vi "fgv_sound_info.vi"(7 "cmd":T2, 8 "error in (no error)":errorcluster caption="error in", 11 "info":T1) -> (0 "error out":errorcluster, 3 "info out":T1)   [LabVIEW 2019]
uses:
  Ctrl/cmd_common.ctl
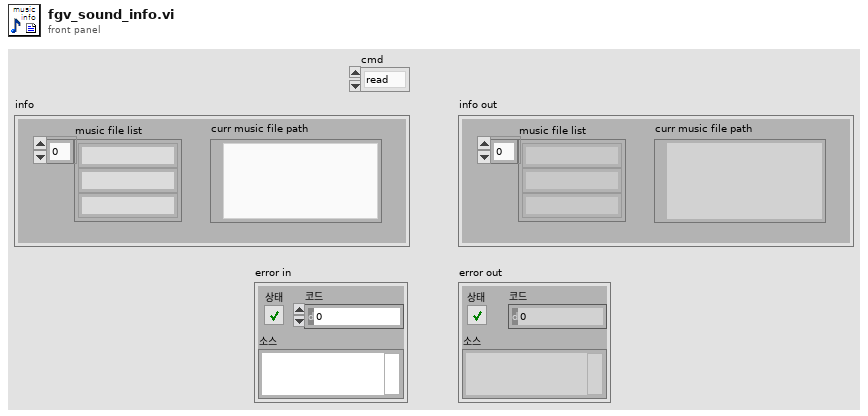
[diagram p1: front panel]
types:
  T1 = cluster{"music file list":string[], "curr music file path":path}
  T2 = typedef "cmd_common.ctl" = enum16{"read", "write"}
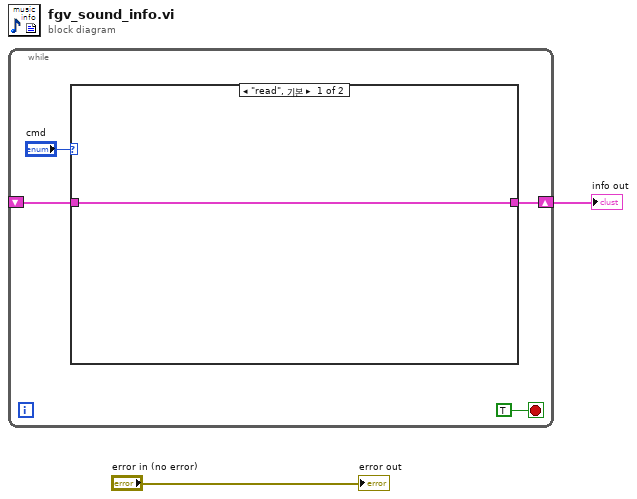
[diagram p0: block diagram]
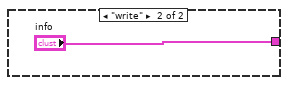
[diagram p2: hidden frame]
diagram:
  n1 = while {
    shift-right: [w4] -> w2
    shift-left: _ -> [w3]
    stop <- TRUE stop-if-true
    n2 = case shown="\"read\", 기본" "cmd" {
      tunnel: [w7 "info"] -> w4
      tunnel: w3 -> [w7 _]
      frame "read", Default {
      }
      frame "write" {
      }
    }
  }
  "info out" <- w2
  "error out" <- "error in (no error)"
